vi "Inverse_kinematic_problem.vi"(1 "Необходимое\nположение\nсхвата":dbl[](array[numeric])) -> (0 "Coords":u32[](array[numeric]))   [LabVIEW 2019]
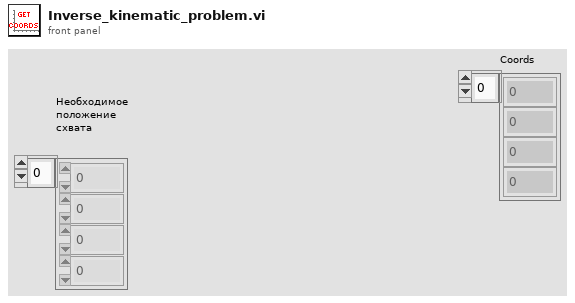
[diagram p1: front panel]
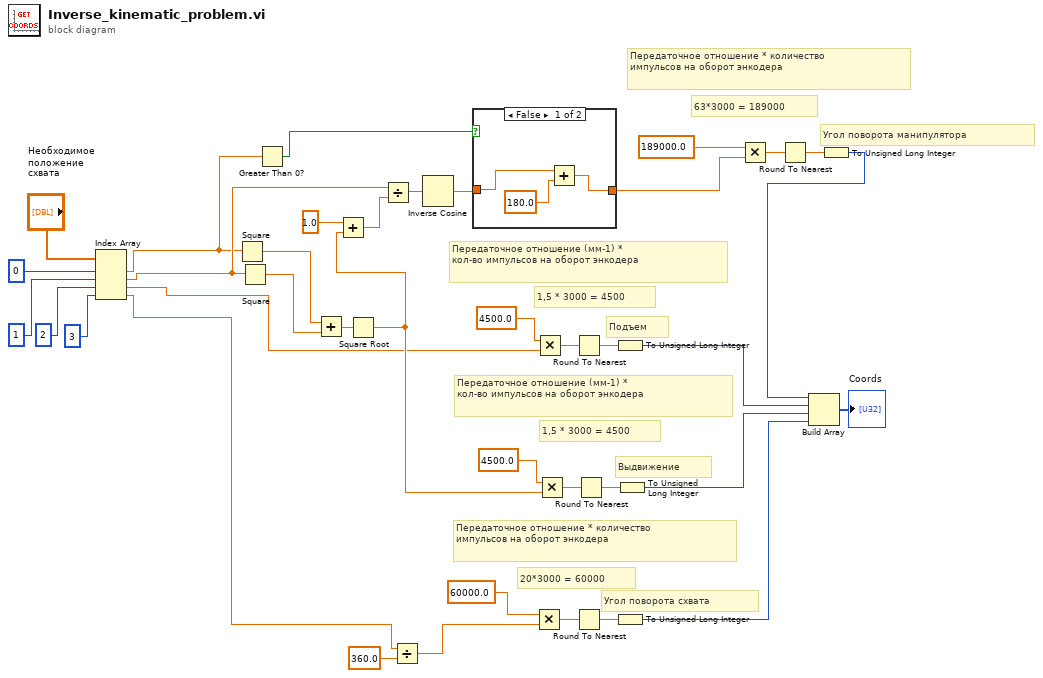
[diagram p0: block diagram]
diagram:
  # "Угол поворота схвата"
  # "Передаточное отношение * количество\nимпульсов на оборот энкодера"
  # "20*3000 = 60000"
  # "Выдвижение"
  # "Передаточное отношение (мм-1) *\nкол-во импульсов на оборот энкодера"
  # "1,5 * 3000 = 4500"
  # "Угол поворота манипулятора"
  # "Подъем"
  # "Передаточное отношение (мм-1) *\nкол-во импульсов на оборот энкодера"
  # "1,5 * 3000 = 4500"
  # "Передаточное отношение * количество\nимпульсов на оборот энкодера"
  # "63*3000 = 189000"
  n1 = Index Array(array="Необходимое\nположение\nсхвата", index #1=0 ("index"), index #2=1 ("index"), index #3=2 ("index"), index #4=3 ("index")) -> (element #1=w1:dbl, element #2=w2:dbl, element #3=w3:dbl, element #4=w4:dbl)
  n2 = Square(x=w1) -> (x^2=w37:dbl)
  n3 = Square(x=w2) -> (x^2=w36:dbl)
  n4 = Greater Than 0?(x=w1) -> (x > 0?=w33:bool)
  n5 = Add(x=w37, y=w36) -> (x+y=w38:dbl)
  n6 = Square Root(x=w38) -> (sqrt(x)=w20:dbl)
  n7 = Add(x=1.0, y=w20) -> (x+y=w34:dbl)
  n8 = Divide(x=w2, y=w34) -> (x/y=w32:dbl)
  n9 = Divide(x=w4, y=360.0) -> (x/y=w10:dbl)
  n10 = Inverse Cosine(1:w32) -> (0:w31:dbl)
  n11 = case shown="False" w33 {
    tunnel: [w39 w42] -> w29
    tunnel: w31 -> [w40 w42]
    frame False {
      n12 = Add(x=w40, y=180.0) -> (x+y=w39:dbl)
    }
    frame True {
    }
  }
  n13 = Multiply(x=60000.0 ("y"), y=w10) -> (x*y=w18:dbl)
  n14 = Multiply(x=4500.0, y=w3) -> (x*y=w24:dbl)
  n15 = Multiply(x=4500.0, y=w20) -> (x*y=w21:dbl)
  n16 = Round To Nearest(number=w24) -> (nearest integer value=w25:dbl)
  n17 = Round To Nearest(number=w18) -> (nearest integer value=w17:dbl)
  n18 = Round To Nearest(number=w21) -> (nearest integer value=w22:dbl)
  n19 = To Unsigned Long Integer(number=w25) -> (unsigned 32bit integer=w15:u32)
  n20 = To Unsigned Long Integer(number=w17) -> (unsigned 32bit integer=w13:u32)
  n21 = To Unsigned Long Integer(number=w22) -> (unsigned 32bit integer=w14:u32)
  n22 = Multiply(x=189000.0 ("y"), y=w29) -> (x*y=w28:dbl)
  n23 = Round To Nearest(number=w28) -> (nearest integer value=w27:dbl)
  n24 = To Unsigned Long Integer(number=w27) -> (unsigned 32bit integer=w16:u32)
  n25 = Build Array(w16, w15, w14, w13) -> (→"Coords":u32[])
